vi "waitForNewWaveforms.vi"(7 "address":string, 8 "error in (no error)":errorcluster) -> (0 "error out":errorcluster, 3 "Newest AI":waveform(dbl)[](array[waveform]))   [LabVIEW 2016]
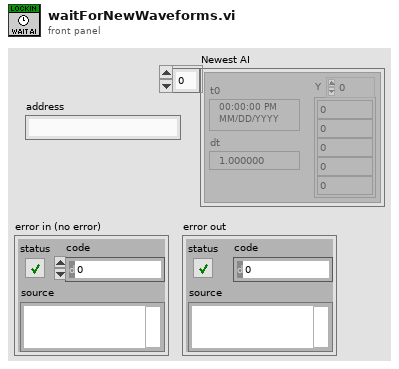
[diagram p1: front panel]
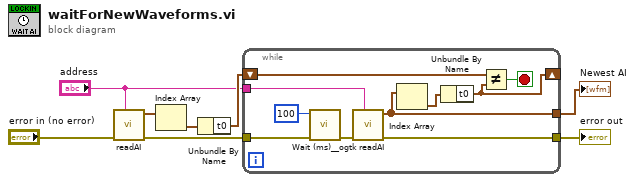
[diagram p0: block diagram]
diagram:
  n1 = call "readAI.vi"("address"="address", "error in (no error)"="error in (no error)") -> ("error out"=w8:errorcluster, "input signal"=w5:waveform(dbl)[])  [unwired: 8 in]
  n2 = Index Array(array=w5) -> (element=w6:waveform(dbl))  [unwired: 1 in]
  n3 = Unbundle By Name(w6) -> ("t0"=w7:timestamp)
  n4 = while {
    shift-right: [w13] -> _
    shift-left: w7 -> [w15]
    tunnel: w8 -> [w16]
    tunnel: [w14] -> w3
    tunnel: "address" -> [w10]
    tunnel: [w9] -> w1
    stop <- w18 stop-if-true
    n5 = call <userlib>:"Wait (ms)__ogtk.vi"("error in (no error)"=w16, "milliseconds to wait"=u32 100) -> ("error out"=w12:errorcluster)  [unwired: 8 in, 1 out]
    n6 = call "readAI.vi"("address"=w10, "error in (no error)"=w12) -> ("error out"=w14:errorcluster, "input signal"=w9:waveform(dbl)[])  [unwired: 8 in]
    n7 = Index Array(array=w9) -> (element=w17:waveform(dbl))  [unwired: 1 in]
    n8 = Unbundle By Name(w17) -> ("t0"=w13:timestamp)
    n9 = Not Equal?(x=w15, y=w13) -> (x != y?=w18:bool)
  }
  "error out" <- w3
  "Newest AI" <- w1
